vi "record_tsv_SC.vi"(5 "logging_on":bool=TRUE, 6 "error in":errorcluster, 7 "subsys_name":string="TargetDAQ", 9 "value":dbl=10.0, 10 "time":timestamp, 11 "var_name":string="VarName") -> (0 "status":bool, 4 "error out":errorcluster)   [LabVIEW 2019]
uses:
  <vilib>/Utility/file.llb/Write Delimited Spreadsheet (string).vi
panel:
  out "file_name":string
  in  "base_dir":string="z:\\e1039_data\\slowcontrol_data"
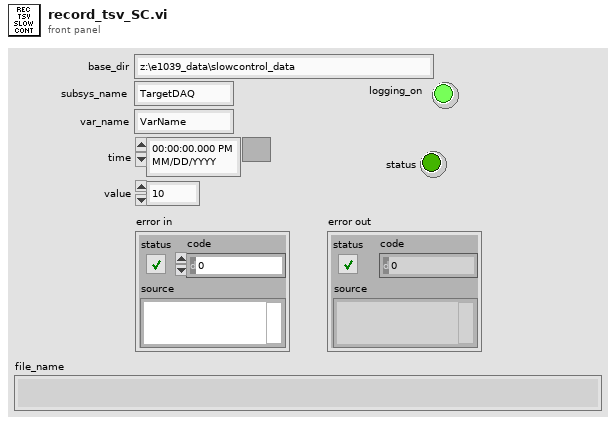
[diagram p1: front panel]
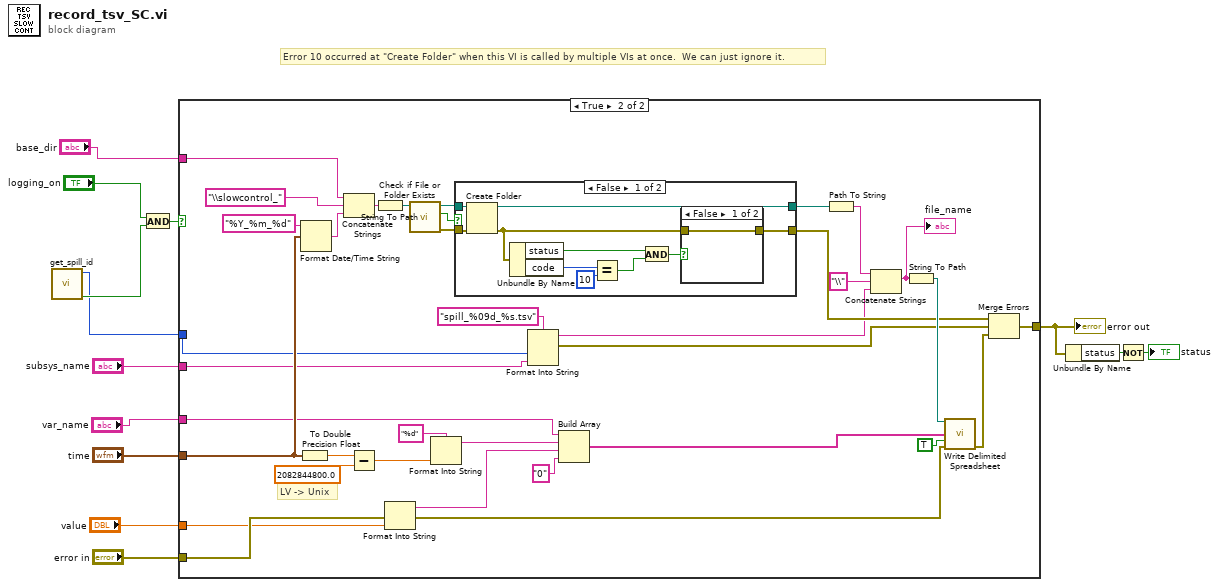
[diagram p0: block diagram]
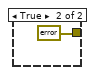
[diagram p3: hidden frame]
diagram:
  # "Error 10 occurred at \"Create Folder\" when this VI is called by multiple VIs at once.  We can just ignore it."
  n1 = call "get_spill_id.vi"() -> ("status"=w5:bool, "spill_id"=w4:i32)  [unwired: 10 in]
  n2 = And(x="logging_on", y=w5) -> (x .and. y?=w7:bool)
  n3 = case shown="True" w7 {
    tunnel: "subsys_name" -> [_ w28]
    tunnel: [w14 w34] -> w10
    tunnel: "time" -> [_ w36]
    tunnel: "error in" -> [w14 w38]
    tunnel: w4 -> [_ w29]
    tunnel: "value" -> [_ w27]
    tunnel: "var_name" -> [_ w25]
    tunnel: "base_dir" -> [_ w23]
    frame False {
    }
    frame True {
      # "LV -> Unix"
      n4 = To Double Precision Float(number=w36) -> (double precision float=w42:dbl)
      n5 = Format Date/Time String(time format string (%c)="%Y_%m_%d", seconds (now)=w36) -> (date/time string=w22:string)  [unwired: 1 in]
      n6 = Concatenate Strings(w23, "\\slowcontrol_", w22) -> (w39:string)
      n7 = Subtract(x=w42, y=2082844800.0) -> (x-y=w16:dbl)
      n8 = String To Path(string=w39) -> (path=w48:path)
      n9 = Format Into String(error in=w38, w27) -> (resulting string=w40:string, error out=w37:errorcluster)  [unwired: 2 in]
      n10 = call <vilib>:"Check if File or Folder Exists.vi"("path"=w48) -> ("error out"=w33:errorcluster, "file or folder exists?"=w47:bool, "dup path"=w45:path)  [unwired: 8 in]
      n11 = Format Into String(format string="%d", w16) -> (resulting string=w26:string)  [unwired: 2 in, 1 out]
      n12 = case shown="False" w47 {
        tunnel: w45 -> [w60 w64]
        tunnel: [w59 w64] -> w46
        tunnel: w33 -> [w58 w63]
        tunnel: [w51 w63] -> w20
        frame False {
          n13 = Create Folder(path (use dialog)=w60, error in=w58) -> (created path=w59:path, error out=w52:errorcluster)  [unwired: 1 in, 1 out]
          n14 = Unbundle By Name(w52) -> ("status"=w55:bool, "code"=w57:i32)
          n15 = Equal?(x=w57, y=10) -> (x = y?=w54:bool)
          n16 = And(x=w55, y=w54) -> (x .and. y?=w53:bool)
          n17 = case shown="False" w53 {
            tunnel: w52 -> [w61 _]
            tunnel: [w61 errorcluster {"status"=FALSE, "code"=0, "source"=""} ("error out")] -> w51
            frame False {
            }
            frame True {
            }
          }
        }
        frame True {
        }
      }
      n18 = Format Into String(format string="spill_%09d_%s.tsv", w29, w28) -> (resulting string=w17:string, error out=w19:errorcluster)  [unwired: 2 in]
      n19 = Build Array(w25, w26, w40, "0" ("element")) -> (w35:string[])
      n20 = Path To String(path=w46) -> (string=w44:string)
      n21 = Concatenate Strings(w44, "\\" ("string"), w17) -> (w49:string)
      "file_name" <- w49
      n22 = String To Path(string=w49) -> (path=w43:path)
      n23 = call-poly <vilib>:"Write Delimited Spreadsheet.vi"("file path (dialog if empty)"=w43, "1D data"=w35, "append to file? (new file:F)"=TRUE, "error in (no error)"=w37) -> ("error out"=w32:errorcluster)  [unwired: 10 in, 1 out]
      n24 = Merge Errors(w20, w19, w32) -> (w34:errorcluster)
    }
  }
  "error out" <- w10
  n25 = Unbundle By Name(w10) -> ("status"=w9:bool)
  n26 = Not(x=w9) -> (.not. x?=→"status":bool)
